vi "Destroy.vi"(8 "error in":errorcluster, 11 "_Rename in":refnum<class "_Rename.lvclass">) -> (0 "error out":errorcluster)   [LabVIEW 2020, in "_Rename.lvlib" / "_Rename.lvclass"]
uses:
  _Rename.lvclass
  <vilib>/Utility/EditLVProj/Edit LVProj.lvlib
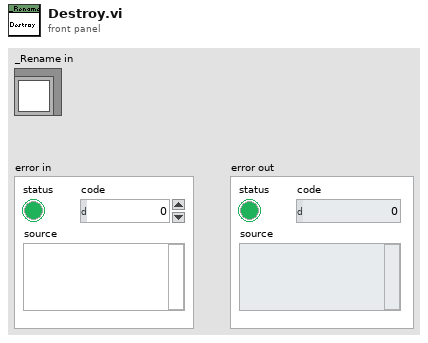
[diagram p1: front panel]
types:
  T1 = typedef "Edit LVProj.lvlib/Library And VI References.ctl" = cluster{"Target Reference":refnum<vi>, "VI References":refnum<vi>[], "Library References":refnum<vi>[]}
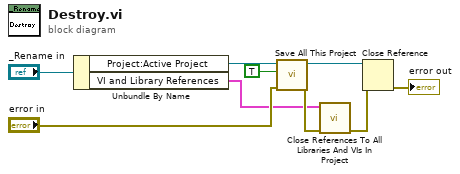
[diagram p0: block diagram]
diagram:
  n1 = Unbundle By Name("_Rename in") -> ("Project:Active Project"=w6:refnum<vi>, "VI and Library References"=w1:T1[])
  n2 = call <vilib>:"Save All This Project.vi"("error in (no error)"="error in", "Exclude Dependencies? (F)"=TRUE, "Project in"=w6) -> ("error out"=w8:errorcluster, "Project out"=w7:refnum<vi>)  [unwired: 7 in]
  n3 = call <vilib>:"Close References To All Libraries And VIs In Project.vi"("error in (no error)"=w8, "VI and Library References"=w1) -> ("error out"=w9:errorcluster)  [unwired: 9 in]
  n4 = Close Reference(reference=w7, error in (no error)=w9) -> (error out=→"error out":errorcluster)
